vi "PI Send.vi"(0 "System no.":i32=1 min=1 step=1, 1 "Error check settings":T1(ring)=enum."Use global settings", 2 "String to send":string, 3 "Attach termination char.?":bool=TRUE, 5 "error in":errorcluster, 7 "Delay before error check (ms)":u32) -> (14 "Controller error":bool, 19 "error out":errorcluster)   [LabVIEW 2020]
doc: "This VI acquires the semaphore for the corresponding system via PI acquire semaphore.vi, sends a string w/o termination character via the selected interface and releases the semaphore via PI release semaphore.vi"
uses:
  Global1.vi
panel:
  # "This vi sends a string w/o termination character via the selected interface."
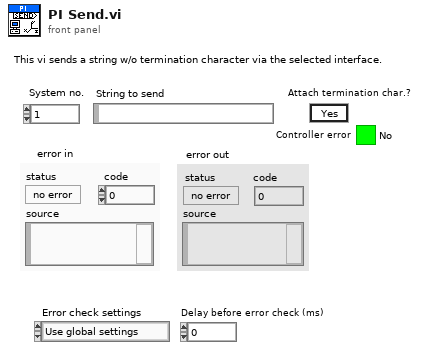
[diagram p1: front panel]
types:
  T1 = enum16{"Disable error check", "Force error check", "Use global settings"}
  T2 = typedef "Semaphore RefNum" = refnum<k1>
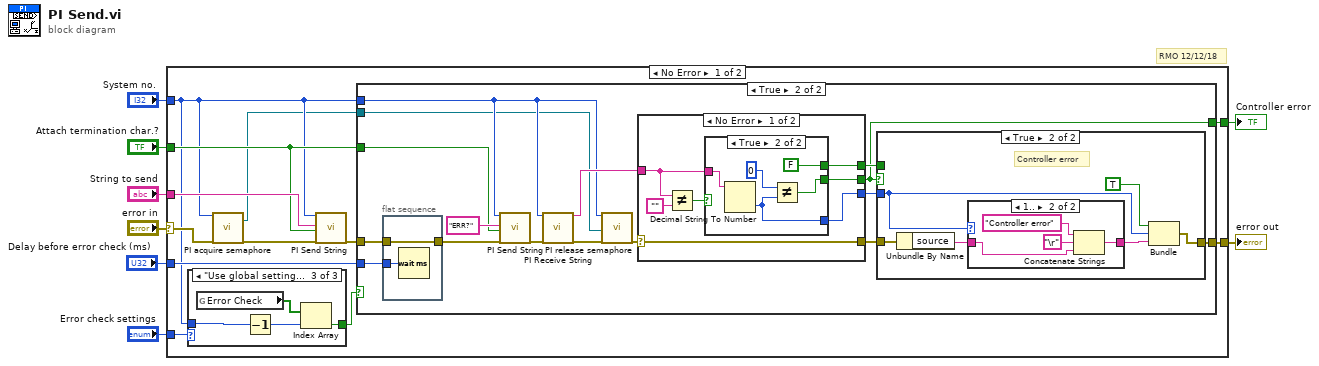
[diagram p0: block diagram]
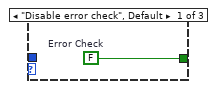
[diagram p2: hidden frame]
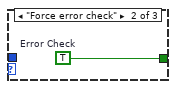
[diagram p3: hidden frame]
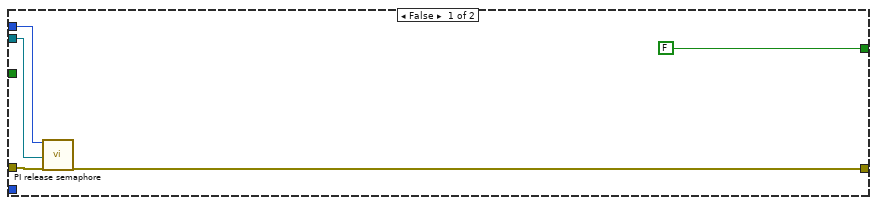
[diagram p4: hidden frame]
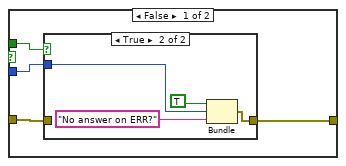
[diagram p5: hidden frame]
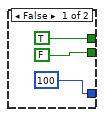
[diagram p8: hidden frame]
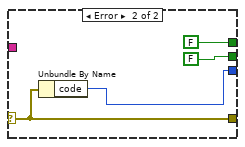
[diagram p9: hidden frame]
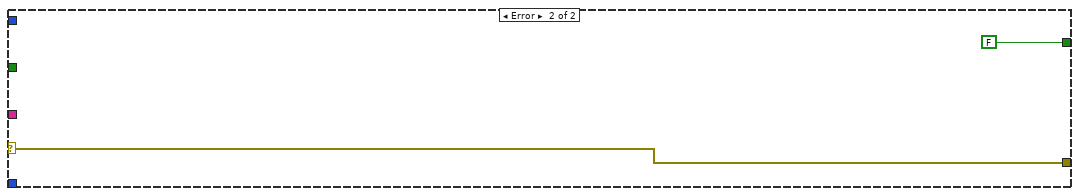
[diagram p10: hidden frame]
diagram:
  # "RMO 12/12/18"
  n1 = case shown="No Error" "error in" {
    selector: "error in" -> [w12 w89]
    tunnel: [w20 w89] -> w3
    tunnel: "String to send" -> [w18 _]
    tunnel: "Attach termination char.?" -> [w17 _]
    tunnel: "System no." -> [w10 _]
    tunnel: [w16 FALSE] -> w6
    tunnel: "Delay before error check (ms)" -> [w15 _]
    tunnel: "Error check settings" -> [w14 _]
    frame No Error {
      n2 = case shown="\"Use global settings\"" w14 {
        tunnel: w10 -> [_ _ w25]
        tunnel: [w21 w22 w23] -> w13
        frame "Disable error check", Default {
          w21 = FALSE  # Error Check
        }
        frame "Force error check" {
          w22 = TRUE  # Error Check
        }
        frame "Use global settings" {
          n3 = global read "Global1.vi" "Error Check"() -> (w26:bool[])
          n4 = Decrement(x=w25) -> (x-1=w24:i32)
          n5 = Index Array(array=w26, index=w24) -> (element=w23:bool)
        }
      }
      n6 = call "PI acquire semaphore.vi"("System no."=w10, "error in"=w12) -> ("semaphore out"=w9:T2, "error out"=w11:errorcluster)  [unwired: 16 out]
      n7 = call "PI Send String.vi"("System no."=w10, "String to send"=w18, "Attach termination char.?"=w17, "error in"=w11) -> ("error out"=w19:errorcluster)  [unwired: 15 out]
      n8 = case shown="True" w13 {
        tunnel: w19 -> [w30 w43]
        tunnel: [w29 w45] -> w20
        tunnel: w10 -> [w28 w35]
        tunnel: w17 -> [_ w39]
        tunnel: [FALSE w44] -> w16
        tunnel: w15 -> [_ w42]
        tunnel: w9 -> [w27 w34]
        frame False {
          n9 = call "PI release semaphore.vi"("System no."=w28, "semaphore"=w27, "error in"=w30) -> ("error out"=w29:errorcluster)  [unwired: 1 in, 15 out]
        }
        frame True {
          n10 = flat-sequence {
            tunnel: w43 -> [w49]
            tunnel: [w49] -> w41
            tunnel: w42 -> [w48]
            frame #0 {
              n11 = Wait (ms)(milliseconds to wait=w48) -> ()  [unwired: 1 out]
            }
          }
          n12 = call "PI Send String.vi"("System no."=w35, "String to send"="ERR?", "Attach termination char.?"=w39, "error in"=w41) -> ("error out"=w37:errorcluster)  [unwired: 15 out]
          n13 = call "PI Receive String.vi"("System no."=w35, "error in"=w37) -> ("String read"=w38:string, "error out"=w36:errorcluster)  [unwired: 1 in, 15 out]
          n14 = call "PI release semaphore.vi"("System no."=w35, "semaphore"=w34, "error in"=w36) -> ("error out"=w33:errorcluster)  [unwired: 1 in, 15 out]
          n15 = case shown="No Error" w33 {
            selector: w33 -> [w70 w85]
            tunnel: w38 -> [w74 _]
            tunnel: [w76 FALSE ("Controller Error")] -> w44
            tunnel: [w75 w86] -> w47
            tunnel: [w71 FALSE ("Controller Error")] -> w46
            tunnel: [w70 w85] -> w32
            frame No Error {
              n16 = Not Equal?(x=w74, y="") -> (x != y?=w73:bool)
              n17 = case shown="True" w73 {
                tunnel: [FALSE w84] -> w76
                tunnel: w74 -> [_ w82]
                tunnel: [100 w81] -> w75
                tunnel: [TRUE FALSE] -> w71
                frame False {
                }
                frame True {
                  n18 = Decimal String To Number(string=w82) -> (number=w81:i32)  [unwired: 3 out]
                  n19 = Not Equal?(x=0, y=w81) -> (x != y?=w84:bool)
                }
              }
            }
            frame Error {
              n20 = Unbundle By Name(w85) -> ("code"=w86:i32)
            }
          }
          n21 = case shown="True" w44 {
            tunnel: w47 -> [w50 w62]
            tunnel: [w52 w64] -> w45
            tunnel: w32 -> [w53 w60]
            tunnel: w46 -> [w51 _]
            frame False {
              n22 = case shown="True" w51 {
                tunnel: w53 -> [w54 _]
                tunnel: [w54 w55] -> w52
                tunnel: w50 -> [_ w57]
                frame False {
                }
                frame True {
                  n23 = Bundle("status"=TRUE, "code"=w57, "No answer on ERR?") -> (w55:cluster{"status":bool, "code":i32, string})  [unwired: 1 out]
                }
              }
            }
            frame True {
              # "Controller error"
              n24 = Unbundle By Name(w60) -> ("source"=w59:string)
              n25 = case shown="1.." w62 {
                tunnel: [w65 w69] -> w61
                tunnel: w59 -> [w65 w67]
                frame ..0 {
                }
                frame 1.. {
                  n26 = Concatenate Strings("Controller error", "\r" ("Substring"), w67) -> (w69:string)
                }
              }
              n27 = Bundle("status"=TRUE, "code"=w62, "source"=w61) -> (w64:errorcluster)  [unwired: 1 out]
            }
          }
        }
      }
    }
    frame Error {
    }
  }
  "error out" <- w3
  "Controller error" <- w6
